vi "MH_AllocateAllHistoBuffer.vi"(10 "NumChan":i32, 11 "HistoLength":i32) -> (3 "Buffer":u32[](array[numeric]))   [LabVIEW 2023]
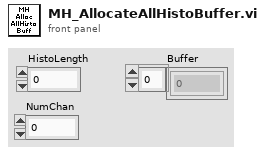
[diagram p1: front panel]
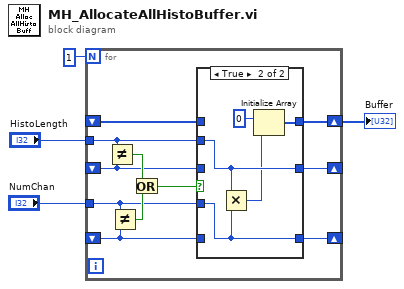
[diagram p0: block diagram]
diagram:
  n1 = for {
    N: 1 -> [_]
    shift-right: [w9] -> _
    shift-left: _ -> [w5]
    tunnel: "HistoLength" -> [w10]
    shift-right: [w15] -> w4
    shift-left: _ -> [w14]
    tunnel: "NumChan" -> [w8]
    shift-right: [w7] -> _
    shift-left: _ -> [w6]
    n2 = Not Equal?(x=w10, y=w5) -> (x != y?=w12:bool)
    n3 = Not Equal?(x=w8, y=w6) -> (x != y?=w13:bool)
    n4 = Or(x=w12, y=w13) -> (x .or. y?=w11:bool)
    n5 = case shown="True" w11 {
      tunnel: [w18 w22] -> w15
      tunnel: w14 -> [w18 _]
      tunnel: w10 -> [_ w21]
      tunnel: [w16 w21] -> w9
      tunnel: w8 -> [_ w20]
      tunnel: [w17 w20] -> w7
      tunnel: w6 -> [w17 _]
      tunnel: w5 -> [w16 _]
      frame False {
      }
      frame True {
        n6 = Multiply(x=w21, y=w20) -> (x*y=w19:i32)
        n7 = Initialize Array(u32 0, w19) -> (w22:u32[])
      }
    }
  }
  "Buffer" <- w4
